vi "avant match.vi"() -> ()   [LabVIEW 2019]
uses:
  <vilib>/Rock Robotics/WPI/SafetyOutput/WPI_SafetyOutputConfigMenu.ctl
  <vilib>/Rock Robotics/SystemInterfaces/DIO/FPGA_DIOChannel.ctl
  <vilib>/Rock Robotics/SystemInterfaces/AI/FPGA_AIChannel.ctl
  <vilib>/Rock Robotics/WPI/ThirdParty/Phoenix-LabVIEW/Motor Controller/Get/CTRE_Phoenix_MotorController_GetQuadratureData.vi
  <vilib>/Rock Robotics/WPI/Solenoid/Deprecated/WPI_SolenoidGetBool.vi
panel:
  out "color sensor":bool
  out "mot lanceur 2":bool
  out "crochet":bool
  out "mot lanceur":bool
  out "mot balayeuse":bool
  out "balayeuse pist":bool
  out "mot bac 2":bool
  out "bac 5":bool
  out "bac 2":bool
  out "bac 1":bool
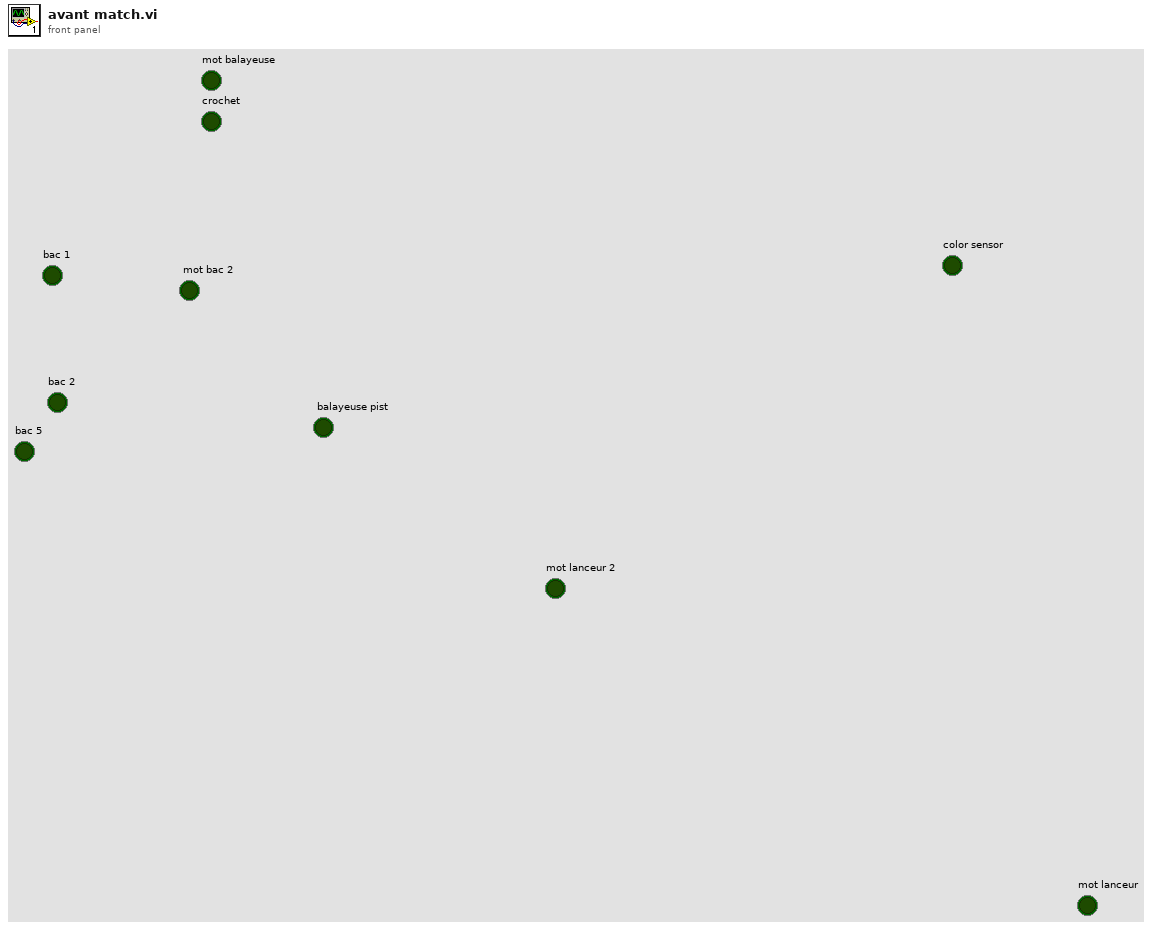
[diagram p1: front panel]
types:
  T1 = typedef "FPGA_AIChannel.ctl" = enum8{"AI 0", "AI 1", "AI 2", "AI 3", "AI MXP 0", "AI MXP 1", "AI MXP 2", "AI MXP 3", "Invalid"}
  T2 = typedef "FPGA_DIOChannel.ctl" = enum8{"DIO 0", "DIO 1", "DIO 2", "DIO 3", "DIO 4", "DIO 5", "DIO 6", "DIO 7", "DIO 8", "DIO 9", "DIO MXP 0", "DIO MXP 1", "DIO MXP 2", "DIO MXP 3", "DIO MXP 4", "DIO MXP 5", "DIO MXP 6", "DIO MXP 7", "DIO MXP 8", "DIO MXP 9", "DIO MXP 10", "DIO MXP 11", "DIO MXP 12", "DIO MXP 13", "DIO MXP 14", "DIO MXP 15", "SPI Port CS1", "SPI Port CS2", "SPI Port CS3", "SPI Port MISO", "SPI Port MOSI", "Invalid"}
  T3 = typedef "WPI_SafetyOutputConfigMenu.ctl" = enum16{"Enable", "Disable"}
  T4 = typedef "WPI_RobotDriveDevRef.ctl" = cluster{"DevStatus":errorcluster, "Motors[]":T5[], "Square Inputs":bool, "Max Output":dbl}
  T5 = typedef "WPI_MotorControlDeviceRef.ctl" = cluster{"DeviceStatus":errorcluster, "Type":T6, "PWM":cluster{"PWM Channel":T7, "DeadBand":T8}, "CAN":cluster{"Device Number":u8, "SetOutput VI Ref":variant, "GetOutput VI Ref":variant, "Enable VI Ref":variant, "Disable VI Ref":variant, "Data":variant}, "Invert":bool, "DIO PWM":cluster{"PWM \"Enable\" Channel":T7, "DIOChannel":T2, "PWM Rate":dbl}}
  T6 = typedef "WPI_MotorControlType.ctl" = enum16{"PWM", "CAN", "DIO PWM"}
  T7 = typedef "FPGA_DIOPWMChannel.ctl" = enum8{"PWM 0", "PWM 1", "PWM 2", "PWM 3", "PWM 4", "PWM 5", "PWM 6", "PWM 7", "PWM 8", "PWM 9", "PWM MXP 0", "PWM MXP 1", "PWM MXP 2", "PWM MXP 3", "PWM MXP 4", "PWM MXP 5", "PWM MXP 6", "PWM MXP 7", "PWM MXP 8", "PWM MXP 9", "Invalid"}
  T8 = typedef "WPI_PWMDeadband.ctl" = cluster{"Name":string, "maxPositivePwm":i32, "minPositivePwm":i32, "centerPwm":i32, "maxNegativePwm":i32, "minNegativePwm":i32, "angularRange":u16}
  T9 = typedef "WPI_AnalogChannelDevRef.ctl" = cluster{"DevStatus":errorcluster, "Analog Channel":T1}
  T10 = typedef "WPI_DigitalInputDevRef.ctl" = cluster{"DevStatus":errorcluster, "DIO Channel":T2}
  T11 = typedef "WPI_SwitchDevRef.ctl" = cluster{"DevStatus":errorcluster, "DIO Channel":T2, "CntIndex":T12, "Normally Closed":bool}
  T12 = typedef "FPGA_CounterCtrSystemIndex.ctl" = enum8{"Ctr 0", "Ctr 1", "Ctr 2", "Ctr 3", "Ctr 4", "Ctr 5", "Ctr 6", "Ctr 7", "Invalid"}
  T13 = typedef "WPI_SolenoidDevRef.ctl" = cluster{"DevStatus":errorcluster, "Pneumatics Control Module":u8, "Forward Solenoid Channel":T14, "Reverse Solenoid Channel":T14}
  T14 = typedef "WPI_SolenoidChannel.ctl" = enum8{"Solenoid 0", "Solenoid 1", "Solenoid 2", "Solenoid 3", "Solenoid 4", "Solenoid 5", "Solenoid 6", "Solenoid 7", "Invalid"}
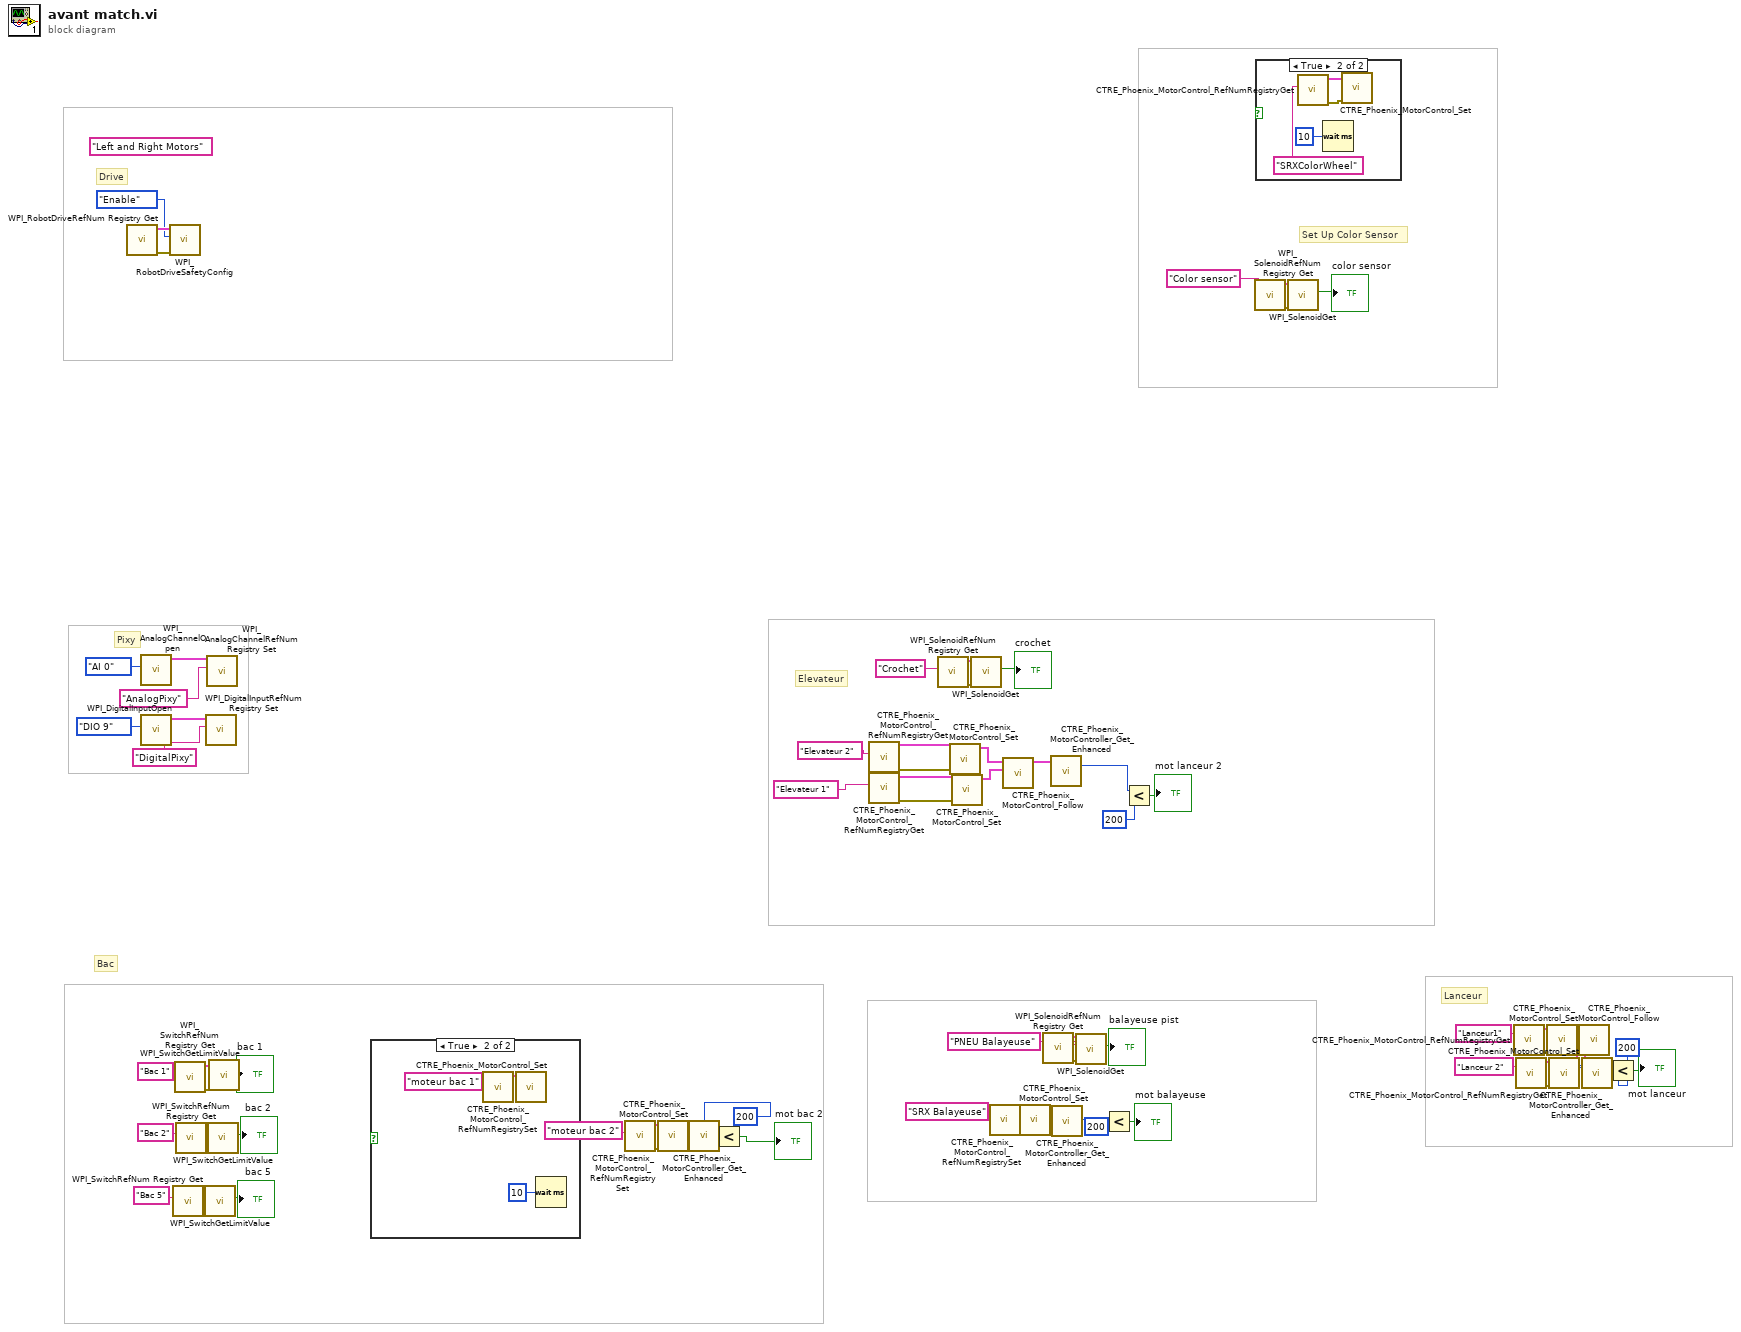
[diagram p0: block diagram]
diagram:
  (unwired) "Left and Right Motors" ("refnum name")
  # "Lanceur"
  # "Set Up Color Sensor"
  # "Pixy"
  # "Bac"
  # "Elevateur"
  # "Drive"
  n1 = call <vilib>:"WPI_RobotDriveRefNum Registry Get.vi"() -> ("error out"=w7:errorcluster, "RobotDriveDevRef"=w6:T4)  [unwired: 10 in]
  n2 = call <vilib>:"WPI_AnalogChannelOpen.vi"("Analog Channel"=FPGA_AIChannel."AI 0") -> ("AIDeviceRef"=w72:T9)  [unwired: 9 in, 1 out]
  n3 = call <vilib>:"WPI_DigitalInputOpen.vi"("DIO Channel"=FPGA_DIOChannel."DIO 9") -> ("DigitalInputDevRef"=w69:T10)  [unwired: 9 in, 1 out]
  n4 = call <vilib>:"WPI_RobotDriveSafetyConfig.vi"("error in (no error)"=w7, "mode"=WPI_SafetyOutputConfigMenu."Enable", "RobotDriveDevRef"=w6) -> ()  [unwired: 7 in, 2 out]
  n5 = call <vilib>:"WPI_SwitchRefNum Registry Get.vi"("refnum name"="Bac 5") -> ("error out"=w62:errorcluster, "SwitchDevRef"=w61:T11)  [unwired: 9 in]
  n6 = call <vilib>:"WPI_SwitchRefNum Registry Get.vi"("refnum name"="Bac 1") -> ("error out"=w58:errorcluster, "SwitchDevRef"=w57:T11)  [unwired: 9 in]
  n7 = call <vilib>:"WPI_SwitchRefNum Registry Get.vi"("refnum name"="Bac 2") -> ("error out"=w60:errorcluster, "SwitchDevRef"=w59:T11)  [unwired: 9 in]
  n8 = call <vilib>:"WPI_SwitchGetLimitValue.vi"("error in (no error)"=w62, "SwitchDevRef"=w61) -> ("Switch Pressed"=→"bac 5":bool)  [unwired: 7 in, 2 out]
  n9 = call <vilib>:"WPI_DigitalInputRefNum Registry Set.vi"("refnum name"="DigitalPixy", "DigitalInputDevRef"=w69) -> ()  [unwired: 8 in, 2 out]
  n10 = call <vilib>:"WPI_AnalogChannelRefNum Registry Set.vi"("refnum name"="AnalogPixy", "AIDeviceRef"=w72) -> ()  [unwired: 8 in, 2 out]
  n11 = call <vilib>:"WPI_SwitchGetLimitValue.vi"("error in (no error)"=w60, "SwitchDevRef"=w59) -> ("Switch Pressed"=→"bac 2":bool)  [unwired: 7 in, 2 out]
  n12 = call <vilib>:"WPI_SwitchGetLimitValue.vi"("error in (no error)"=w58, "SwitchDevRef"=w57) -> ("Switch Pressed"=→"bac 1":bool)  [unwired: 7 in, 2 out]
  n13 = case shown="True" {
    selector: _ -> [_ _]
    frame False {
    }
    frame True {
      n14 = call <vilib>:"CTRE_Phoenix_MotorControl_RefNumRegistrySet.vi"("refnum name"="moteur bac 1") -> ("PhoenixMotorControlDevRef"=w75:T5)  [unwired: 9 in, 1 out]
      n15 = call <vilib>:"CTRE_Phoenix_MotorControl_Set.vi"("PhoenixMotorControlDevRef"=w75) -> ()  [unwired: 9 in, 2 out]
      n16 = Wait (ms)(milliseconds to wait=u32 10) -> ()  [unwired: 1 out]
    }
  }
  n17 = call <vilib>:"CTRE_Phoenix_MotorControl_RefNumRegistrySet.vi"("refnum name"="moteur bac 2") -> ("error out"=w56:errorcluster, "PhoenixMotorControlDevRef"=w55:T5)  [unwired: 9 in]
  n18 = call <vilib>:"CTRE_Phoenix_MotorControl_Set.vi"("error in (no error)"=w56, "PhoenixMotorControlDevRef"=w55) -> ("error out"=w49:errorcluster, "PhoenixMotorControlDevRef"=w50:T5)  [unwired: 8 in]
  n19 = call-poly <vilib>:"CTRE_Phoenix_MotorController_Get_Enhanced.vi"("PhoenixMotorControlDevRef"=w50, "error in"=w49) -> ("Quadrature Position"=w48:i32)  [unwired: 10 in, 3 out]
  n20 = Less?(x=w48, y=200) -> (x < y?=→"mot bac 2":bool)
  n21 = call <vilib>:"CTRE_Phoenix_MotorControl_RefNumRegistryGet.vi"("refnum name"="Elevateur 2") -> ("error out"=w19:errorcluster, "PhoenixMotorControlDevRef"=w18:T5)  [unwired: 9 in]
  n22 = call <vilib>:"CTRE_Phoenix_MotorControl_RefNumRegistryGet.vi"("refnum name"="Elevateur 1") -> ("error out"=w16:errorcluster, "PhoenixMotorControlDevRef"=w17:T5)  [unwired: 9 in]
  n23 = call <vilib>:"WPI_SolenoidRefNum Registry Get.vi"("refnum name"="Crochet") -> ("error out"=w21:errorcluster, "SolenoidDevRef"=w22:T13)  [unwired: 9 in]
  n24 = call <vilib>:"CTRE_Phoenix_MotorControl_Set.vi"("error in (no error)"=w19, "PhoenixMotorControlDevRef"=w18) -> ("PhoenixMotorControlDevRef"=w15:T5)  [unwired: 8 in, 1 out]
  n25 = call <vilib>:"CTRE_Phoenix_MotorControl_Set.vi"("error in (no error)"=w16, "PhoenixMotorControlDevRef"=w17) -> ("PhoenixMotorControlDevRef"=w14:T5)  [unwired: 8 in, 1 out]
  n26 = call-poly <vilib>:"WPI_SolenoidGet.vi"("error in (no error)"=w21, "SolenoidDevRef"=w22) -> ("Value"=→"crochet":bool)  [unwired: 7 in, 2 out]
  n27 = call <vilib>:"CTRE_Phoenix_MotorControl_RefNumRegistrySet.vi"("refnum name"="SRX Balayeuse") -> ("error out"=w41:errorcluster, "PhoenixMotorControlDevRef"=w40:T5)  [unwired: 9 in]
  n28 = call <vilib>:"CTRE_Phoenix_MotorControl_Follow.vi"("Master Controller to Follow"=w14, "PhoenixMotorControlDevRef"=w15) -> ("PhoenixMotorControlDevRef"=w13:T5)  [unwired: 8 in, 1 out]
  n29 = call <vilib>:"CTRE_Phoenix_MotorControl_Set.vi"("error in (no error)"=w41, "PhoenixMotorControlDevRef"=w40) -> ("PhoenixMotorControlDevRef"=w37:T5)  [unwired: 8 in, 1 out]
  n30 = call <vilib>:"WPI_SolenoidRefNum Registry Get.vi"("refnum name"="PNEU Balayeuse") -> ("error out"=w45:errorcluster, "SolenoidDevRef"=w44:T13)  [unwired: 9 in]
  n31 = call-poly <vilib>:"CTRE_Phoenix_MotorController_Get_Enhanced.vi"("PhoenixMotorControlDevRef"=w13) -> ("Quadrature Position"=w10:i32)  [unwired: 11 in, 3 out]
  n32 = call-poly <vilib>:"CTRE_Phoenix_MotorController_Get_Enhanced.vi"("PhoenixMotorControlDevRef"=w37) -> ("Quadrature Position"=w39:i32)  [unwired: 11 in, 3 out]
  n33 = call-poly <vilib>:"WPI_SolenoidGet.vi"("error in (no error)"=w45, "SolenoidDevRef"=w44) -> ("Value"=→"balayeuse pist":bool)  [unwired: 7 in, 2 out]
  n34 = Less?(x=w39, y=200) -> (x < y?=→"mot balayeuse":bool)
  n35 = Less?(x=w10, y=200) -> (x < y?=→"mot lanceur 2":bool)
  n36 = call <vilib>:"WPI_SolenoidRefNum Registry Get.vi"("refnum name"="Color sensor") -> ("error out"=w3:errorcluster, "SolenoidDevRef"=w4:T13)  [unwired: 9 in]
  n37 = case shown="True" {
    selector: _ -> [_ _]
    frame False {
    }
    frame True {
      n38 = call <vilib>:"CTRE_Phoenix_MotorControl_RefNumRegistryGet.vi"("refnum name"="SRXColorWheel") -> ("error out"=w78:errorcluster, "PhoenixMotorControlDevRef"=w79:T5)  [unwired: 9 in]
      n39 = Wait (ms)(milliseconds to wait=u32 10) -> ()  [unwired: 1 out]
      n40 = call <vilib>:"CTRE_Phoenix_MotorControl_Set.vi"("error in (no error)"=w78, "PhoenixMotorControlDevRef"=w79) -> ()  [unwired: 8 in, 2 out]
    }
  }
  n41 = call-poly <vilib>:"WPI_SolenoidGet.vi"("error in (no error)"=w3, "SolenoidDevRef"=w4) -> ("Value"=→"color sensor":bool)  [unwired: 7 in, 2 out]
  n42 = call <vilib>:"CTRE_Phoenix_MotorControl_RefNumRegistryGet.vi"("refnum name"="Lanceur1") -> ("error out"=w34:errorcluster, "PhoenixMotorControlDevRef"=w35:T5)  [unwired: 9 in]
  n43 = call <vilib>:"CTRE_Phoenix_MotorControl_RefNumRegistryGet.vi"("refnum name"="Lanceur 2") -> ("error out"=w31:errorcluster, "PhoenixMotorControlDevRef"=w32:T5)  [unwired: 9 in]
  n44 = call <vilib>:"CTRE_Phoenix_MotorControl_Set.vi"("error in (no error)"=w34, "PhoenixMotorControlDevRef"=w35) -> ("PhoenixMotorControlDevRef"=w26:T5)  [unwired: 8 in, 1 out]
  n45 = call <vilib>:"CTRE_Phoenix_MotorControl_Set.vi"("error in (no error)"=w31, "PhoenixMotorControlDevRef"=w32) -> ("PhoenixMotorControlDevRef"=w25:T5)  [unwired: 8 in, 1 out]
  n46 = call <vilib>:"CTRE_Phoenix_MotorControl_Follow.vi"("Master Controller to Follow"=w25, "PhoenixMotorControlDevRef"=w26) -> ("PhoenixMotorControlDevRef"=w24:T5)  [unwired: 8 in, 1 out]
  n47 = call-poly <vilib>:"CTRE_Phoenix_MotorController_Get_Enhanced.vi"("PhoenixMotorControlDevRef"=w24) -> ("Quadrature Position"=w28:i32)  [unwired: 11 in, 3 out]
  n48 = Less?(x=w28, y=200) -> (x < y?=→"mot lanceur":bool)
